vi "Create InconsistentList.vi"(8 "error in (no error)":errorcluster, 11 "initial allocated size":i32=128) -> (0 "error out":errorcluster, 3 "inconsistent list":refnum<class "NI_Robotics_InconsistentList.lvclass">)   [LabVIEW 2017, in "NI_Robotics_InconsistentList.lvclass"]
uses:
  <vilib>/robotics/Navigation/shared/InconsistentList/NI_Robotics_InconsistentList.lvclass
  <vilib>/robotics/Navigation/shared/MapNode/AbstractDstarNode/NI_Robotics_AbstractDstarNode.lvclass
  <vilib>/robotics/Navigation/shared/InconsistentList/NI_Robotics_InconsistentList.lvclass/NI_Robotics_InconsistentList.ctl
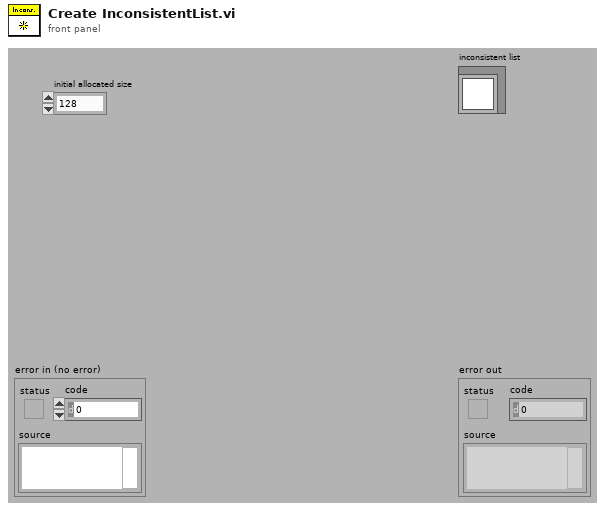
[diagram p1: front panel]
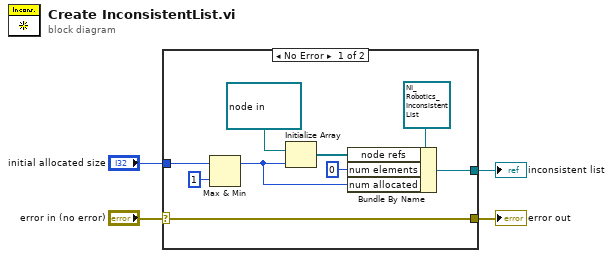
[diagram p0: block diagram]
diagram:
  n1 = case shown="No Error" "error in (no error)" {
    selector: "error in (no error)" -> [w13 w14]
    tunnel: [w13 w14] -> w3
    tunnel: "initial allocated size" -> [w6 _]
    tunnel: [w8 _] -> w1
    frame No Error {
      n2 = Max & Min(x=w6, y=1) -> (max(x,y)=w5:i32)  [unwired: 1 out]
      n3 = Initialize Array(refnum<data-value> refnum ("node ref"), w5) -> (w9:refnum<data-value>[])
      n4 = Bundle By Name(cluster=refnum<class "NI_Robotics_InconsistentList.lvclass"> refnum ("NI_Robotics_InconsistentList in"), "node refs"=w9, "num elements"=0, "num allocated"=w5) -> (w8:refnum<class "NI_Robotics_InconsistentList.lvclass">)
    }
    frame Error {
    }
  }
  "error out" <- w3
  "inconsistent list" <- w1
